vi "[RT] Global Stop Handler.vi"(4 "Reset?":bool, 8 "Error In":errorcluster, 9 "Initiate Stop?":bool) -> (2 "Error Out":errorcluster, 3 "Stop?":bool)   [LabVIEW 2017]
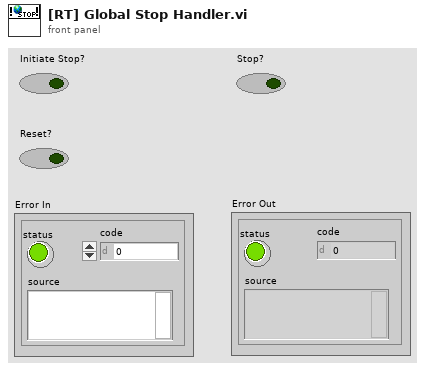
[diagram p1: front panel]
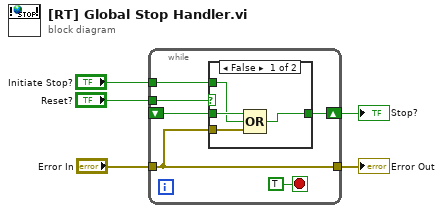
[diagram p0: block diagram]
diagram:
  n1 = while {
    tunnel: "Error In" -> [w6]
    shift-right: [w10] -> w4
    shift-left: _ -> [w11]
    tunnel: [w6] -> w3
    tunnel: "Reset?" -> [w8]
    tunnel: "Initiate Stop?" -> [w7]
    stop <- TRUE stop-if-true
    n2 = case shown="False" w8 {
      tunnel: w11 -> [w15 _]
      tunnel: [w14 FALSE] -> w10
      tunnel: w6 -> [w13 _]
      tunnel: w7 -> [w12 _]
      frame False {
        n3 = Compound Arithmetic op=OR(w15, w12, w13) -> (w14:bool)
      }
      frame True {
      }
    }
  }
  "Error Out" <- w3
  "Stop?" <- w4
